vi "TE Help Guide.vi"() -> ()   [LabVIEW 2014]
panel:
  out "Steps":picture
  in  "Step":i32=1
  out "Current Step":i32
  in  "Forward":bool
  in  "Back":bool
  in  "Boolean":bool
  # "/ 4"
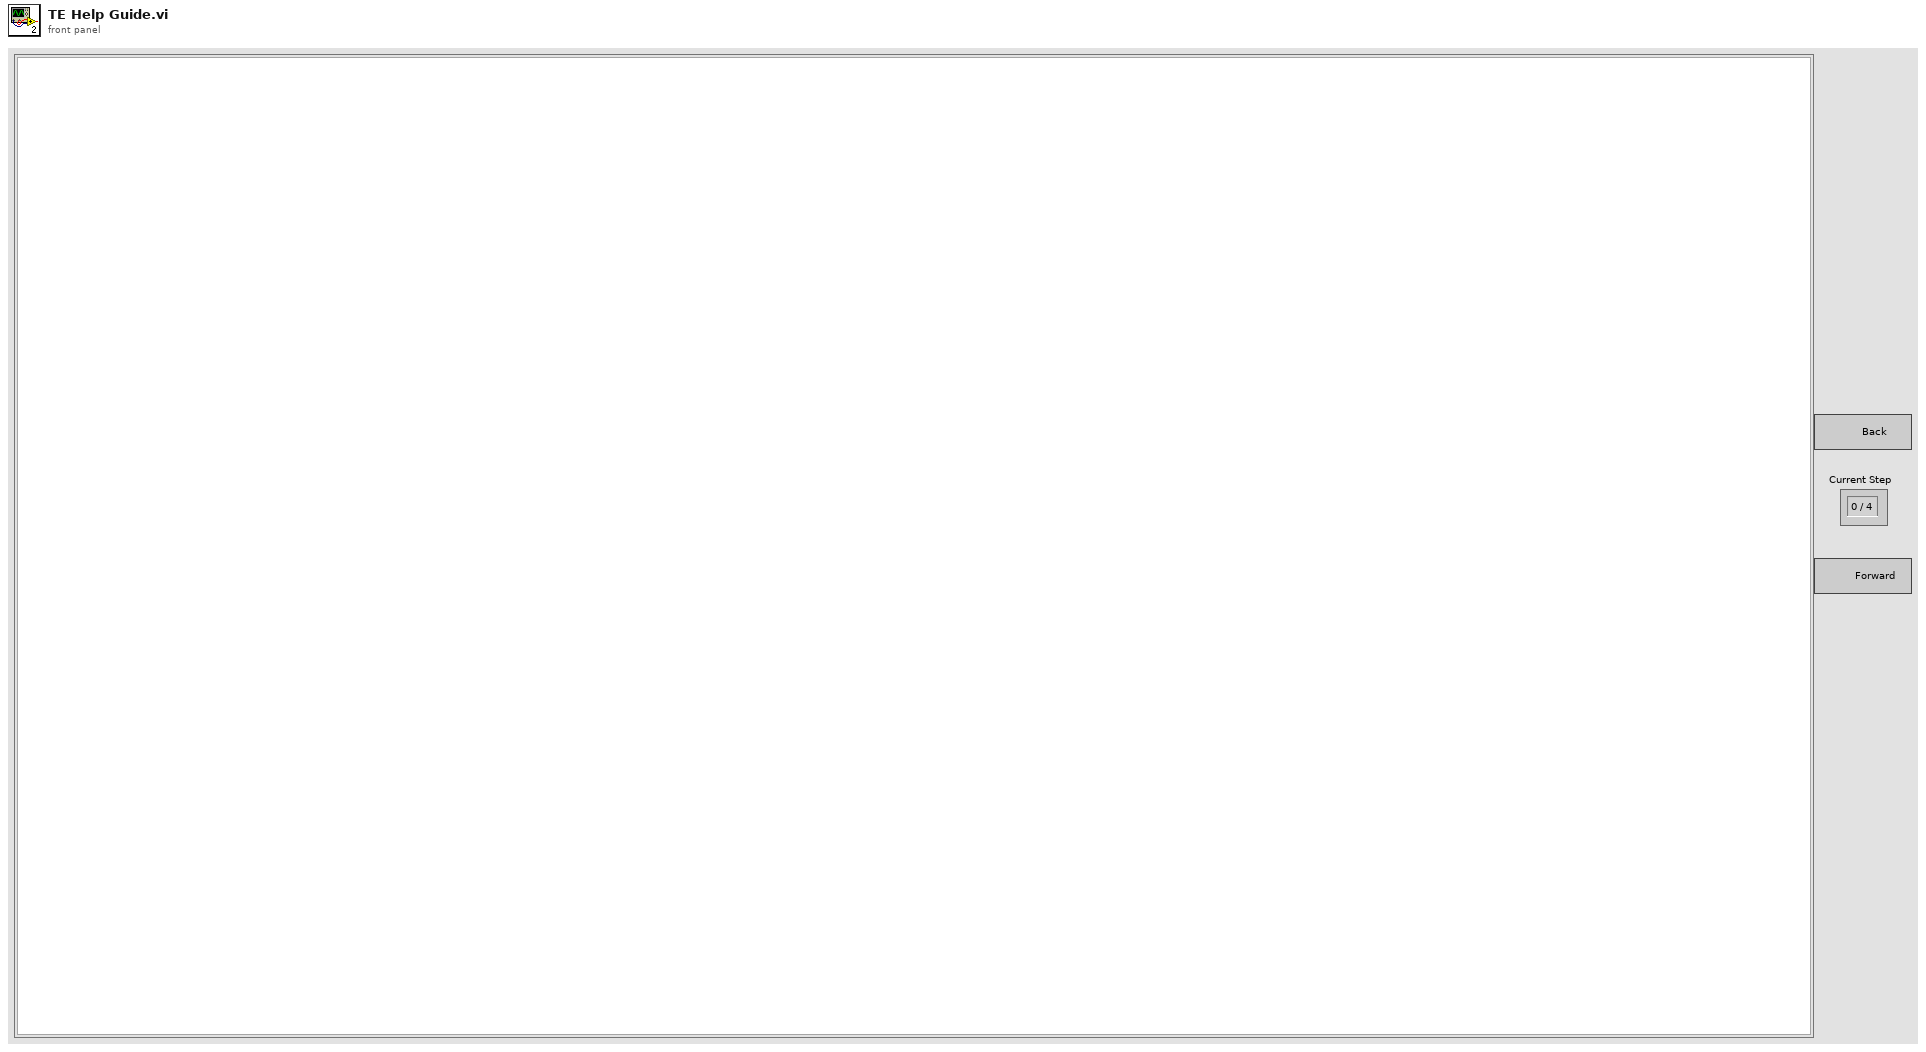
[diagram p1: front panel]
types:
  T1 = typedef "imagedata.ctl" = cluster{"image type":i32, "image depth":i32, "image":u8[], "mask":u8[], "colors":u32[], "Rectangle":cluster{"left":i16, "top":i16, "right":i16, "bottom":i16}}
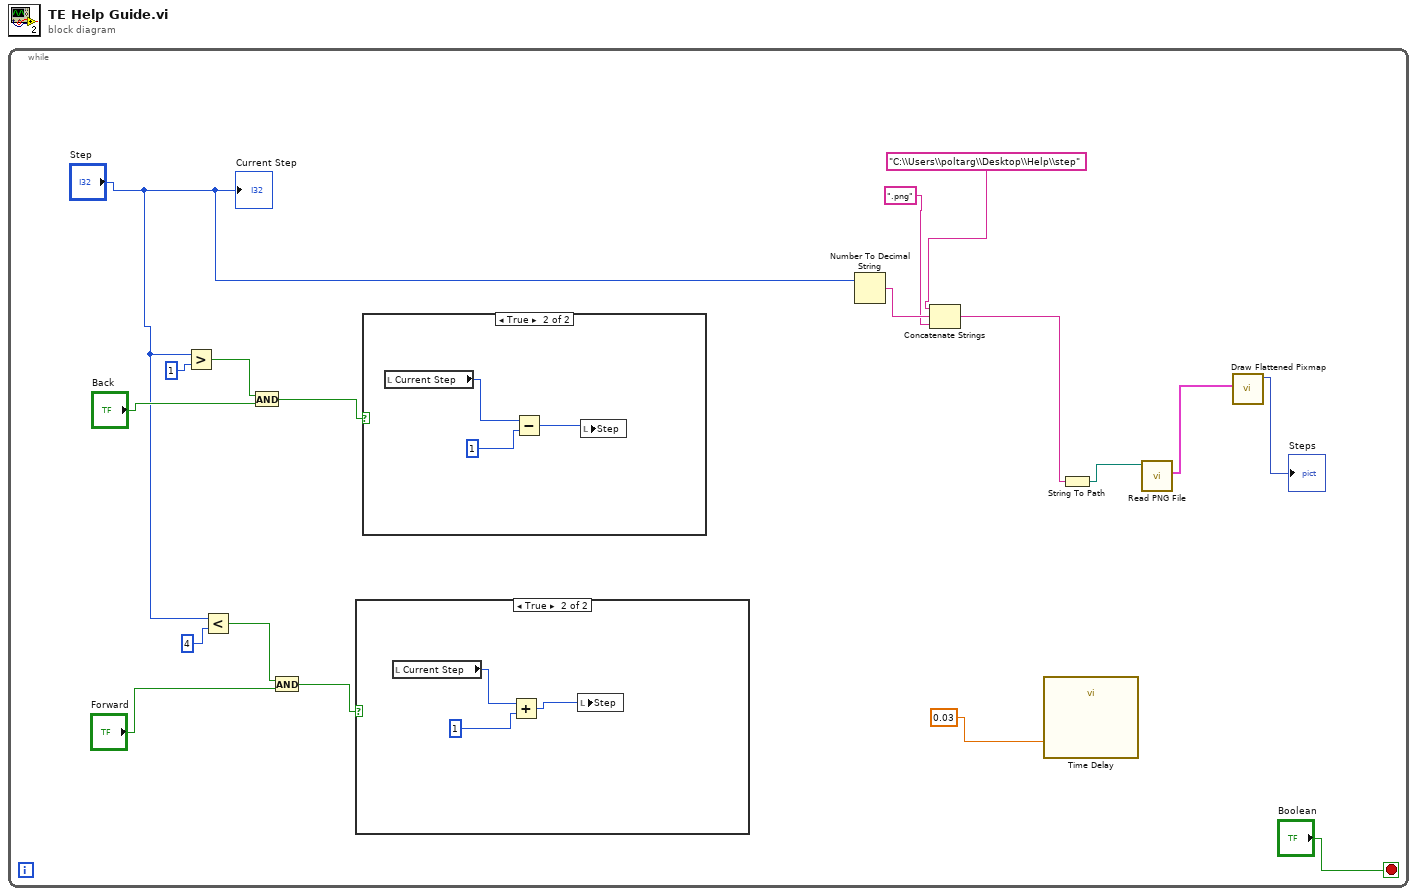
[diagram p0: block diagram]
diagram:
  n1 = while {
    stop <- "Boolean" stop-if-true
    n2 = Greater?(x="Step", y=1) -> (0:w17:bool)
    n3 = Less?(x="Step", y=4) -> (x < y?=w13:bool)
    n4 = And(x=w17, y="Back") -> (x .and. y?=w15:bool)
    n5 = And(x=w13, y="Forward") -> (x .and. y?=w11:bool)
    n6 = case shown="True" w11 {
      frame False {
      }
      frame True {
        n7 = local read "Current Step"() -> (w21:i32)
        n8 = Add(x=w21, y=1) -> (x+y=w19:i32)
        n9 = local write "Step"(w19) -> ()
      }
    }
    n10 = case shown="True" w15 {
      frame False {
      }
      frame True {
        n11 = local read "Current Step"() -> (w23:i32)
        n12 = Subtract(x=w23, y=1) -> (x-y=w22:i32)
        n13 = local write "Step"(w22) -> ()
      }
    }
    n14 = Number To Decimal String(number="Step") -> (decimal integer string=w5:string)  [unwired: 1 in]
    n15 = Concatenate Strings("C:\\Users\\poltarg\\Desktop\\Help\\step", w5, ".png") -> (w3:string)
    n16 = call "Time Delay"("Delay Time (s)"=0.03) -> ()  [unwired: 10 in, 1 out]
    n17 = String To Path(string=w3) -> (path=w8:path)
    n18 = call <vilib>:"Read PNG File.vi"("path to PNG file"=w8) -> ("image data"=w9:T1)  [unwired: 8 in, 2 out]
    n19 = call <vilib>:"Draw Flattened Pixmap.vi"("image data"=w9) -> ("new picture"=→"Steps":picture)  [unwired: 8 in]
    "Current Step" <- "Step"
  }
